vi "Reverse Solver.vi"() -> ()   [LabVIEW 2024]
uses:
  Utility/Universal Utility/TypeDefs_Utility/Cluster_Row-Column.ctl
  Problem-06_Guard Gallivant/ENUM_Direction.ctl
  ff658be3-2798-4a74-9d79-f8928b27ea4f.vi
  5419a5d6-7369-4808-a98a-c8c449d136e9.vi
  138d44c1-2659-4550-9a6a-4fb55107cb8a.vi
  <vilib>/Utility/error.llb/Trim Whitespace.vi
  <vilib>/Utility/error.llb/Trim Whitespace One-Sided.vi
panel:
  out "Num Keypad me":string[](array[string])
  out "R1 Kepad me":string[](array[string])
  out "R2 Kepad me":string[](array[string])
  out "R3 Kepad me":string[](array[string])
  out "Num Keypad":string[](array[string])
  out "R1 Kepad":string[](array[string])
  out "R2 Kepad":string[](array[string])
  out "R3 Kepad":string[](array[string])
  in  "User String":string
  # "<v<A>>^AvA^A<vA<AA>>^AAvA<^A>AAvA^A<vA>^AA<A>A<v<A>A>^AAAvA<^A>A"
  # "v<<A>>^AvA^Av<<A>>^AAv<A<A>>^AAvAA^<A>Av<A^>AA<A>Av<A<A>>^AAA<Av>A^A"
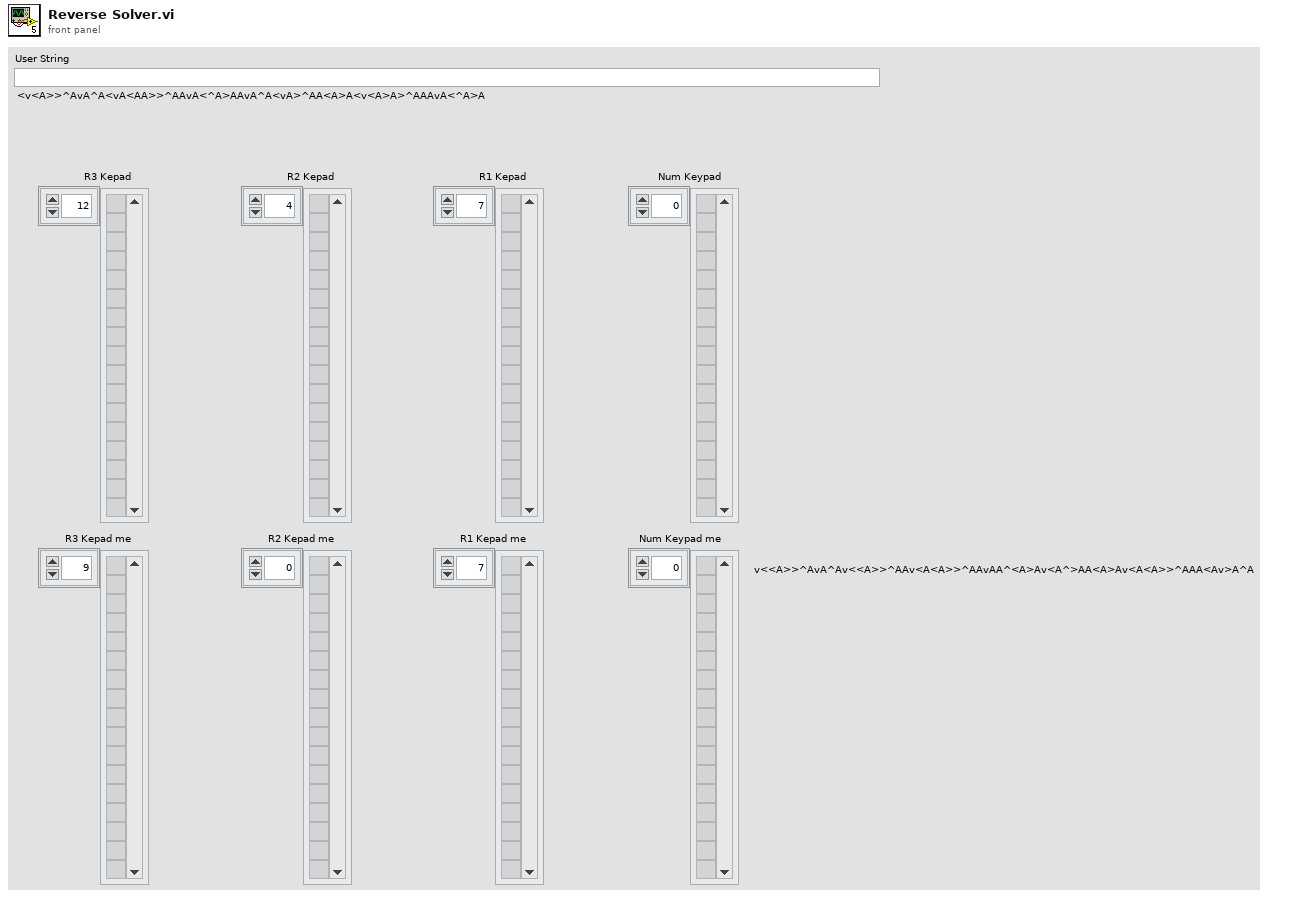
[diagram p1: front panel]
types:
  T1 = typedef "Cluster_Row-Column.ctl" = cluster{"R":i32, "C":i32}
  T2 = typedef "ENUM_Direction.ctl" = enum16{"Up;-1,0", "Right;0,1", "Down;1,0", "Left;0,-1"}
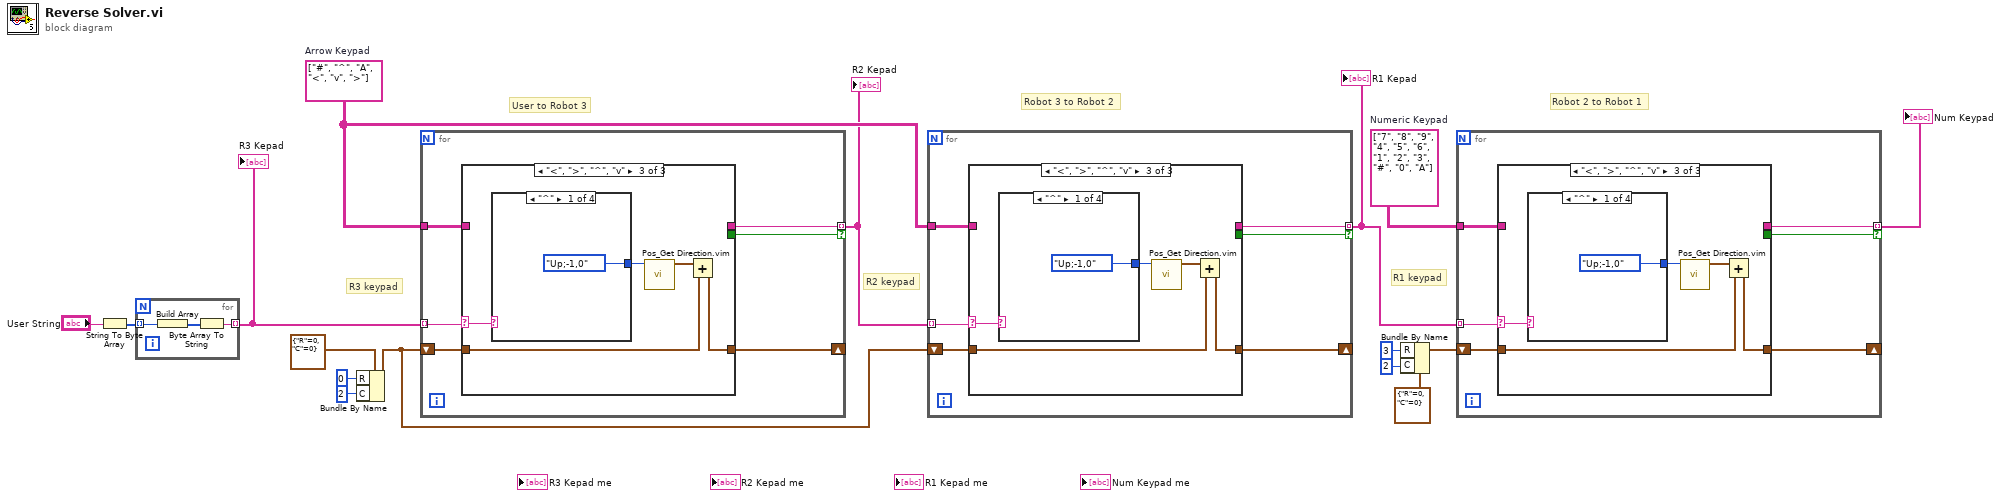
[diagram p0: block diagram]
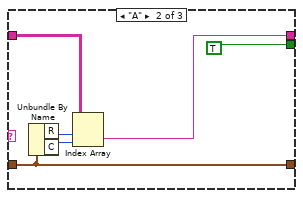
[diagram p3: hidden frame]
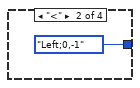
[diagram p4: hidden frame]
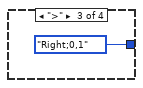
[diagram p5: hidden frame]
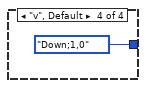
[diagram p6: hidden frame]
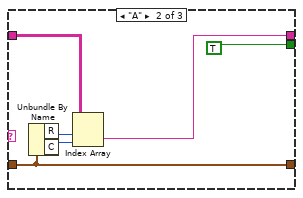
[diagram p8: hidden frame]
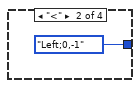
[diagram p9: hidden frame]
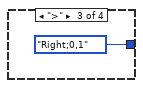
[diagram p10: hidden frame]
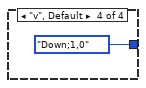
[diagram p11: hidden frame]
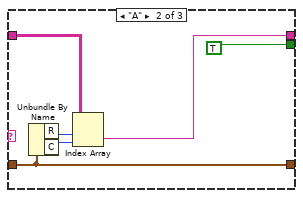
[diagram p13: hidden frame]
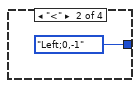
[diagram p14: hidden frame]
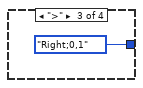
[diagram p15: hidden frame]
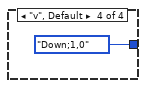
[diagram p16: hidden frame]
diagram:
  w10 = string[][] [["#", "^", "A"], ["<", "v", ">"]]  # Arrow Keypad
  w9 = string[][] [["7", "8", "9"], ["4", "5", "6"], ["1", "2", "3"], ["#", "0", "A"]]  # Numeric Keypad
  # "R1 keypad"
  # "R2 keypad"
  # "R3 keypad"
  # "Robot 2 to Robot 1"
  # "Robot 3 to Robot 2"
  # "User to Robot 3"
  n1 = String To Byte Array(string="User String") -> (unsigned byte array=w16:u8[])
  n2 = for {
    tunnel: w16 -> [w19] mode=indexing
    tunnel: [w17] -> w14 mode=indexing
    n3 = Build Array(w19) -> (w18:u8[])
    n4 = Byte Array To String(unsigned byte array=w18) -> (string=w17:string)
  }
  "R3 Kepad" <- w14
  n5 = Bundle By Name(cluster=T1 {"R"=0, "C"=0} ("Position"), "R"=0, "C"=2) -> (w6:T1)
  n6 = for {
    tunnel: w14 -> [w24] mode=indexing
    tunnel: w10 -> [w25]
    shift-right: [w20] -> _
    shift-left: w6 -> [w23]
    tunnel: [w22] -> w3 mode=indexing if=w21
    n7 = case shown="\"<\", \">\", \"^\", \"v\"" w24 {
      selector: w24 -> [_ _ w33]
      tunnel: w25 -> [_ w32 _]
      tunnel: w23 -> [w26 w27 w35]
      tunnel: [_ w29 _] -> w22
      tunnel: [_ TRUE _] -> w21
      tunnel: [w26 w27 w34] -> w20
      frame Default {
      }
      frame "A" {
        n8 = Unbundle By Name(w27) -> ("R"=w30:i32, "C"=w31:i32)
        n9 = Index Array(array=w32, index (row)=w30, index (col)=w31) -> (element=w29:string)
      }
      frame "<", ">", "^", "v" {
        n10 = case shown="\"^\"" w33 {
          tunnel: [ENUM_Direction."Up;-1,0" ("Direction") ENUM_Direction."Left;0,-1" ("Direction") ENUM_Direction."Right;0,1" ("Direction") ENUM_Direction."Down;1,0" ("Direction")] -> w37
          frame "^" {
          }
          frame "<" {
          }
          frame ">" {
          }
          frame "v", Default {
          }
        }
        n11 = call "Pos_Get Direction.vim"("Direction"=w37) -> ("Position"=w36:T1)  [unwired: 10 in]
        n12 = Add(x=w36, y=w35) -> (x+y=w34:T1)
      }
    }
  }
  "R2 Kepad" <- w3
  n13 = for {
    tunnel: w3 -> [w46] mode=indexing
    tunnel: w10 -> [w47]
    shift-right: [w42] -> _
    shift-left: w6 -> [w45]
    tunnel: [w44] -> w2 mode=indexing if=w43
    n14 = case shown="\"<\", \">\", \"^\", \"v\"" w46 {
      selector: w46 -> [_ _ w55]
      tunnel: w47 -> [_ w54 _]
      tunnel: w45 -> [w48 w49 w57]
      tunnel: [_ w51 _] -> w44
      tunnel: [_ TRUE _] -> w43
      tunnel: [w48 w49 w56] -> w42
      frame Default {
      }
      frame "A" {
        n15 = Unbundle By Name(w49) -> ("R"=w52:i32, "C"=w53:i32)
        n16 = Index Array(array=w54, index (row)=w52, index (col)=w53) -> (element=w51:string)
      }
      frame "<", ">", "^", "v" {
        n17 = case shown="\"^\"" w55 {
          tunnel: [ENUM_Direction."Up;-1,0" ("Direction") ENUM_Direction."Left;0,-1" ("Direction") ENUM_Direction."Right;0,1" ("Direction") ENUM_Direction."Down;1,0" ("Direction")] -> w59
          frame "^" {
          }
          frame "<" {
          }
          frame ">" {
          }
          frame "v", Default {
          }
        }
        n18 = call "Pos_Get Direction.vim"("Direction"=w59) -> ("Position"=w58:T1)  [unwired: 10 in]
        n19 = Add(x=w58, y=w57) -> (x+y=w56:T1)
      }
    }
  }
  "R1 Kepad" <- w2
  n20 = Bundle By Name(cluster=T1 {"R"=0, "C"=0} ("Position"), "R"=3, "C"=2) -> (w5:T1)
  n21 = for {
    tunnel: w2 -> [w68] mode=indexing
    tunnel: w9 -> [w69]
    shift-right: [w64] -> _
    shift-left: w5 -> [w67]
    tunnel: [w66] -> w1 mode=indexing if=w65
    n22 = case shown="\"<\", \">\", \"^\", \"v\"" w68 {
      selector: w68 -> [_ _ w77]
      tunnel: w69 -> [_ w76 _]
      tunnel: w67 -> [w70 w71 w79]
      tunnel: [_ w73 _] -> w66
      tunnel: [_ TRUE _] -> w65
      tunnel: [w70 w71 w78] -> w64
      frame Default {
      }
      frame "A" {
        n23 = Unbundle By Name(w71) -> ("R"=w74:i32, "C"=w75:i32)
        n24 = Index Array(array=w76, index (row)=w74, index (col)=w75) -> (element=w73:string)
      }
      frame "<", ">", "^", "v" {
        n25 = case shown="\"^\"" w77 {
          tunnel: [ENUM_Direction."Up;-1,0" ("Direction") ENUM_Direction."Left;0,-1" ("Direction") ENUM_Direction."Right;0,1" ("Direction") ENUM_Direction."Down;1,0" ("Direction")] -> w81
          frame "^" {
          }
          frame "<" {
          }
          frame ">" {
          }
          frame "v", Default {
          }
        }
        n26 = call "Pos_Get Direction.vim"("Direction"=w81) -> ("Position"=w80:T1)  [unwired: 10 in]
        n27 = Add(x=w80, y=w79) -> (x+y=w78:T1)
      }
    }
  }
  "Num Keypad" <- w1
